vi "LED_rand_wait.vi"(5 "FPGA I/O In":refnum<k21>="IO Module\\D0 0", 6 "Randomly generated testpulse separation input (20 ns ticks)":u32=50000, 7 "Testpulser On/Off":bool, 10 "Testpulse Time Delay (20 ns ticks)":u32=15, 11 "Testpulse duration (20 ns ticks)":u32=1) -> (1 "Is Test Pulse?":bool, 3 "Get New Value":bool)   [LabVIEW 2012]
uses:
  <vilib>/rvi/eio/common/nirviEmuTemplateMethod_errors.vi
  <vilib>/eio/EIONode/EIONode.xnode
panel:
  out "Separation distance counter":u32
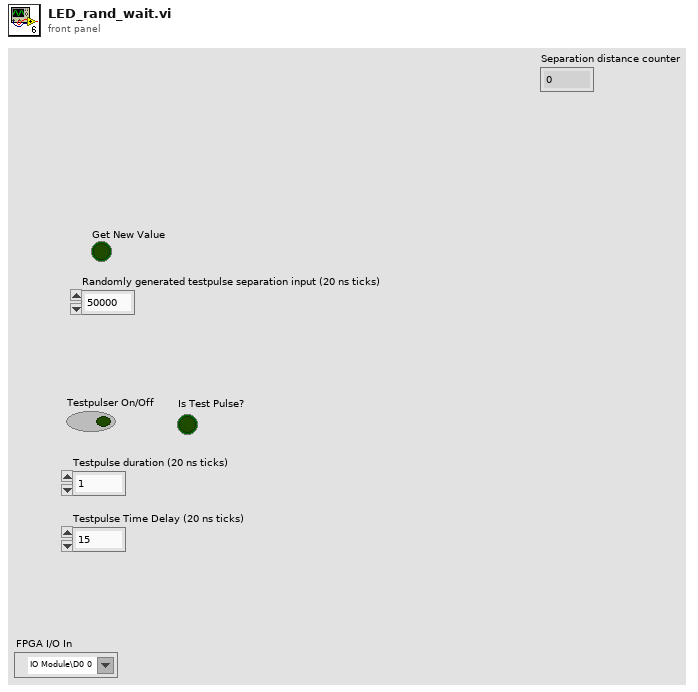
[diagram p1: front panel]
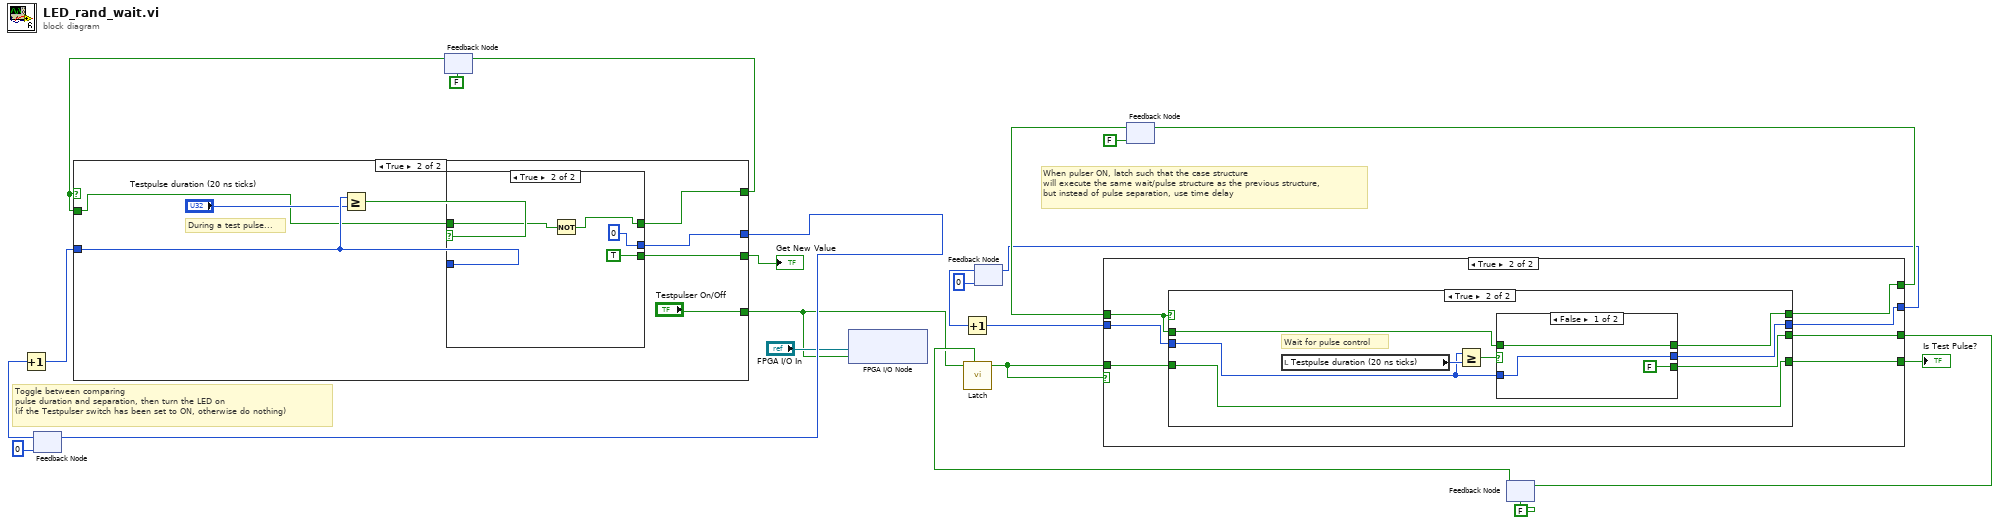
[diagram p0: block diagram]
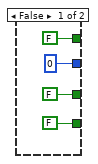
[diagram p2: hidden frame]
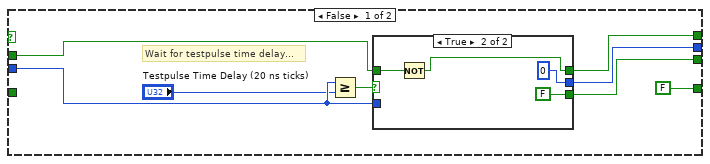
[diagram p3: hidden frame]
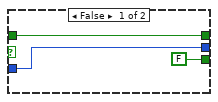
[diagram p4: hidden frame]
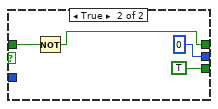
[diagram p5: hidden frame]
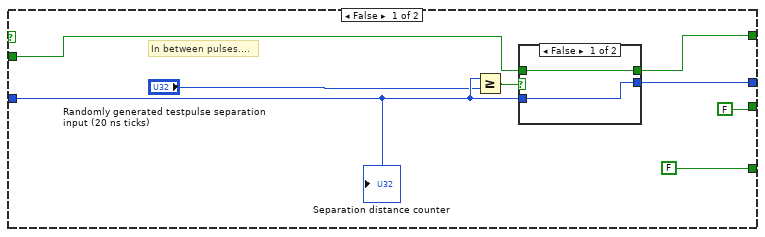
[diagram p6: hidden frame]
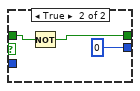
[diagram p7: hidden frame]
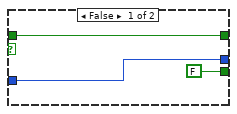
[diagram p8: hidden frame]
diagram:
  # "Toggle between comparing \npulse duration and separation, then turn the LED on\n(if the Testpulser switch has been set to ON, otherwise do nothing)"
  # "When pulser ON, latch such that the case structure\nwill execute the same wait/pulse structure as the previous structure, \nbut instead of pulse separation, use time delay"
  n1 = feedback #1(u32 0) -> (w7:u32)
  n2 = Increment(x=w7) -> (x+1=w4:u32)
  n3 = feedback #2(FALSE) -> (w10:bool)
  n4 = case shown="True" w10 {
    tunnel: w4 -> [w27 w40]
    tunnel: [w30 w42] -> w8
    tunnel: [w29 w43] -> w18
    tunnel: [FALSE ("IO Module\\D0 0") "Testpulser On/Off"] -> w1
    tunnel: w10 -> [w25 w37]
    tunnel: [FALSE w36] -> w3
    frame False {
      # "In between pulses...."
      n5 = Greater Or Equal?(x=w27, y="Randomly generated testpulse separation input (20 ns ticks)") -> (x >= y?=w26:bool)
      n6 = case shown="False" w26 {
        tunnel: [w32 u32 0] -> w30
        tunnel: w27 -> [w32 _]
        tunnel: [w31 w34] -> w29
        tunnel: w25 -> [w31 w33]
        frame False {
        }
        frame True {
          n7 = Not(x=w33) -> (.not. x?=w34:bool)
        }
      }
      "Separation distance counter" <- w27
    }
    frame True {
      # "During a test pulse..."
      n8 = Greater Or Equal?(x=w40, y="Testpulse duration (20 ns ticks)") -> (x >= y?=w39:bool)
      n9 = case shown="True" w39 {
        tunnel: w40 -> [w46 _]
        tunnel: [w45 w50] -> w43
        tunnel: [w46 u32 0] -> w42
        tunnel: w37 -> [w45 w48]
        tunnel: [FALSE TRUE] -> w36
        frame False {
        }
        frame True {
          n10 = Not(x=w48) -> (.not. x?=w50:bool)
        }
      }
    }
  }
  "Get New Value" <- w3
  n11 = feedback-in #1(w8) -> ()
  n12 = feedback-in #2(w18) -> ()
  n13 = xnode "FPGA I/O Node"("I/O Item"=w1, "FPGA I/O In"="FPGA I/O In") -> ()  [unwired: 1 out]
  n14 = feedback #3(u32 0) -> (w12:u32)
  n15 = Increment(x=w12) -> (x+1=w13:u32)
  n16 = feedback #4(FALSE) -> (w16:bool)
  n17 = feedback #5(FALSE) -> (w21:bool)
  n18 = call "Latch.vi"("Reset"=w21, "Input"=w1) -> ("Output"=w22:bool)  [unwired: 9 in]
  n19 = case shown="True" w22 {
    tunnel: w22 -> [_ w56]
    tunnel: [FALSE w58] -> w5
    tunnel: w13 -> [_ w59]
    tunnel: [u32 0 w57] -> w14
    tunnel: w16 -> [_ w61]
    tunnel: [FALSE w60] -> w17
    tunnel: [FALSE w55] -> w20
    frame False {
    }
    frame True {
      n20 = case shown="True" w61 {
        tunnel: w61 -> [w68 w81]
        tunnel: [w67 w80] -> w60
        tunnel: w59 -> [w64 w82]
        tunnel: [FALSE w78] -> w58
        tunnel: [w65 w79] -> w57
        tunnel: w56 -> [_ w78]
        tunnel: [w62 w77] -> w55
        frame False {
          # "Wait for testpulse time delay..."
          n21 = Greater Or Equal?(x=w64, y="Testpulse Time Delay (20 ns ticks)") -> (x >= y?=w69:bool)
          n22 = case shown="True" w69 {
            tunnel: w68 -> [w72 w76]
            tunnel: [w72 w75] -> w67
            tunnel: [w71 u32 0] -> w65
            tunnel: w64 -> [w71 _]
            tunnel: [FALSE FALSE] -> w62
            frame False {
            }
            frame True {
              n23 = Not(x=w76) -> (.not. x?=w75:bool)
            }
          }
        }
        frame True {
          # "Wait for pulse control"
          n24 = local read "Testpulse duration (20 ns ticks)"() -> (w84:u32)
          n25 = Greater Or Equal?(x=w82, y=w84) -> (x >= y?=w83:bool)
          n26 = case shown="False" w83 {
            tunnel: w82 -> [w86 _]
            tunnel: w81 -> [w87 w90]
            tunnel: [w87 w89] -> w80
            tunnel: [w86 u32 0] -> w79
            tunnel: [FALSE TRUE] -> w77
            frame False {
            }
            frame True {
              n27 = Not(x=w90) -> (.not. x?=w89:bool)
            }
          }
        }
      }
    }
  }
  "Is Test Pulse?" <- w5
  n28 = feedback-in #3(w14) -> ()
  n29 = feedback-in #4(w17) -> ()
  n30 = feedback-in #5(w20) -> ()
